vi "test_save_2.vi"() -> ()   [LabVIEW 2016]
panel:
  out "4":i32
  out "3":i32
  out "2":i32
  out "1":i32
  out "4":string
  out "положение 4":i32
  out "3":string
  out "положение 3":i32
  in  "Numeric 4":i32
  in  "Numeric 3":i32
  out "2":string
  out "положение 2":i32
  in  "Numeric 2":i32
  out "положение":i32
  in  "Numeric":i32
  in  "stop":bool
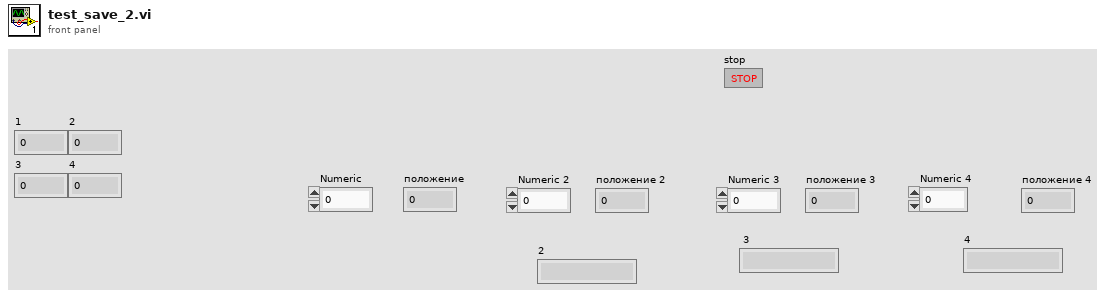
[diagram p1: front panel]
types:
  T1 = enum16{"open", "replace", "create", "open or create", "replace or create", "replace or create with confirmation"}
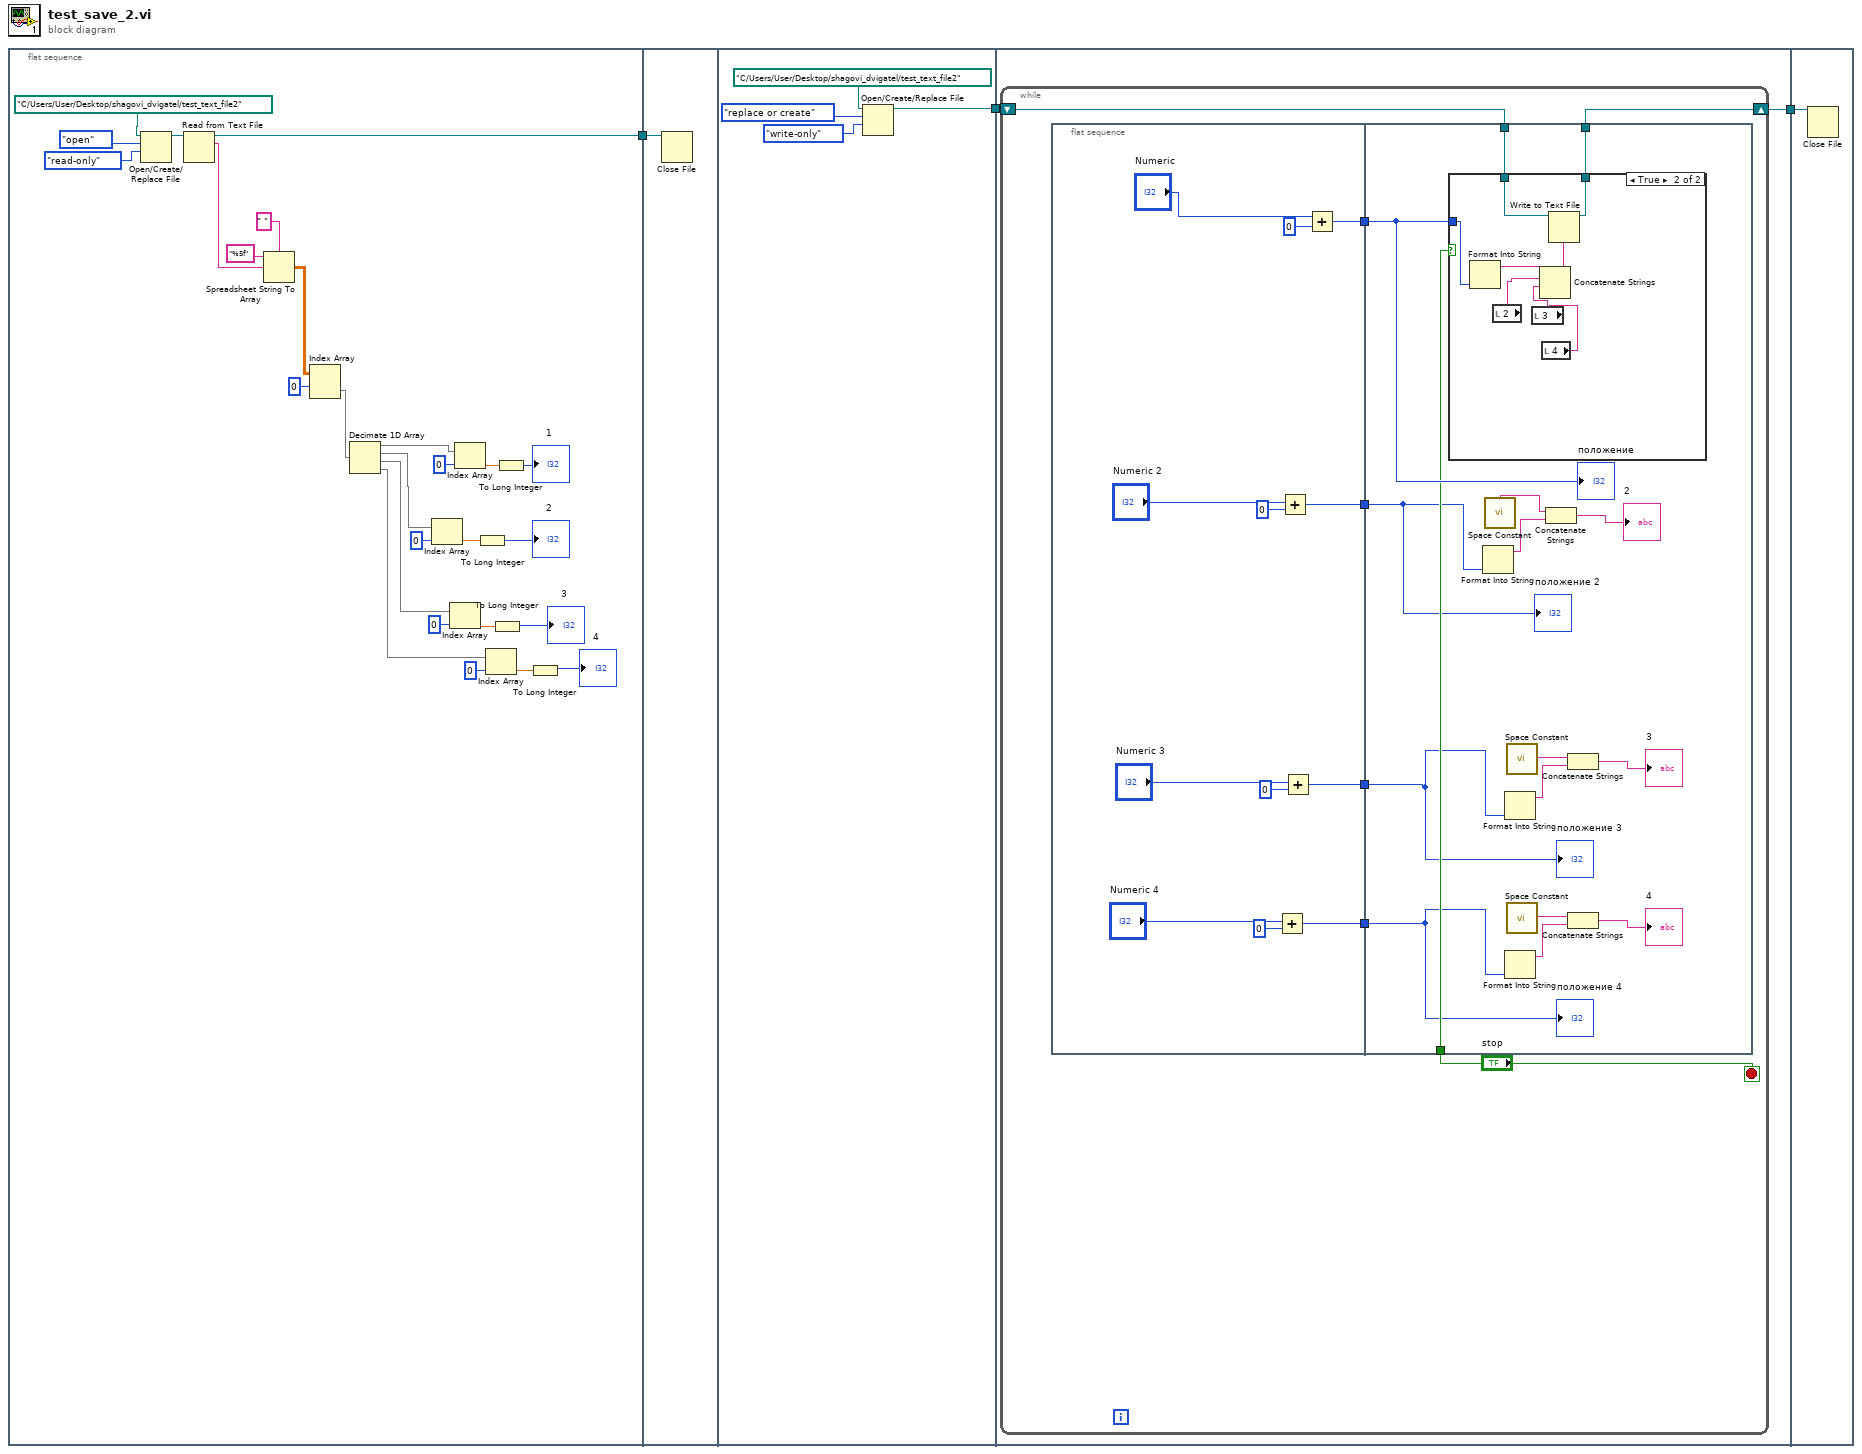
[diagram p0: block diagram]
diagram:
  n1 = flat-sequence {
    tunnel: [w26] -> w3
    tunnel: w3 -> [w31]
    tunnel: [w32] -> w1
    tunnel: [w37] -> w2
    tunnel: w1 -> [w36]
    tunnel: w2 -> [w82]
    frame #0 {
      n2 = Open/Create/Replace File(file path (use dialog)=path "C:/Users/User/Desktop/shagovi_dvigatel/test_text_file2", operation (0:open)=T1."open", access (0:read/write)=enum16{"read/write", "read-only", "write-only"}."read-only") -> (refnum out=w27:refnum<file>)  [unwired: 3 in, 2 out]
      n3 = Read from Text File(file (use dialog)=w27) -> (refnum out=w26:refnum<file>, text=w24:string)  [unwired: 3 in, 2 out]
      n4 = Spreadsheet String To Array(delimiter (Tab)=" ", format string="%5f", spreadsheet string=w24) -> (array=w22:dbl[][])  [unwired: 1 in]
      n5 = Index Array(array=w22, index (row)=0 ("index")) -> (element=w20:dbl[])  [unwired: 1 in]
      n6 = Decimate 1D Array(w20) -> (w12:dbl[], w14:dbl[], w16:dbl[], w19:dbl[])
      n7 = Index Array(array=w14, index=0) -> (element=w9:dbl)
      n8 = Index Array(array=w16, index=0) -> (element=w10:dbl)
      n9 = Index Array(array=w12, index=0) -> (element=w8:dbl)
      n10 = To Long Integer(number=w9) -> (32bit integer=→"2":i32)
      n11 = Index Array(array=w19, index=0) -> (element=w11:dbl)
      n12 = To Long Integer(number=w10) -> (32bit integer=→"3":i32)
      n13 = To Long Integer(number=w8) -> (32bit integer=→"1":i32)
      n14 = To Long Integer(number=w11) -> (32bit integer=→"4":i32)
    }
    frame #1 {
      n15 = Close File(refnum=w31) -> ()  [unwired: 1 in, 2 out]
    }
    frame #2 {
      n16 = Open/Create/Replace File(file path (use dialog)=path "C:/Users/User/Desktop/shagovi_dvigatel/test_text_file2", operation (0:open)=T1."replace or create", access (0:read/write)=enum16{"read/write", "read-only", "write-only"}."write-only") -> (refnum out=w32:refnum<file>)  [unwired: 3 in, 2 out]
    }
    frame #3 {
      n17 = while {
        shift-right: [w44] -> w37
        shift-left: w36 -> [w43]
        stop <- "stop" stop-if-true
        n18 = flat-sequence {
          tunnel: [w55] -> w42
          tunnel: [w53] -> w40
          tunnel: [w46] -> w39
          tunnel: [w45] -> w38
          tunnel: [w72] -> w44
          tunnel: w43 -> [w71]
          tunnel: w42 -> [w70]
          tunnel: "stop" -> [w69]
          tunnel: w40 -> [w68]
          tunnel: w39 -> [w60]
          tunnel: w38 -> [w59]
          frame #0 {
            n19 = Add(x="Numeric 4", y=0) -> (x+y=w46:i32)
            n20 = Add(x="Numeric 2", y=0) -> (x+y=w53:i32)
            n21 = Add(x="Numeric 3", y=0) -> (x+y=w45:i32)
            n22 = Add(x="Numeric", y=0) -> (x+y=w55:i32)
          }
          frame #1 {
            n23 = case shown="True" w69 {
              tunnel: w71 -> [w73 w81]
              tunnel: [w73 w80] -> w72
              tunnel: w70 -> [_ w79]
              frame False {
              }
              frame True {
                n24 = Format Into String(w79) -> (resulting string=w78:string)  [unwired: 3 in, 1 out]
                n25 = local read "2"() -> (w77:string)
                n26 = local read "3"() -> (w75:string)
                n27 = local read "4"() -> (w74:string)
                n28 = Concatenate Strings(w78, w77, w75, w74) -> (w76:string)
                n29 = Write to Text File(file (use dialog)=w81, text=w76) -> (refnum out=w80:refnum<file>)  [unwired: 2 in, 2 out]
              }
            }
            n30 = Format Into String(w68) -> (resulting string=w65:string)  [unwired: 3 in, 1 out]
            n31 = call <vilib>:"Space Constant.vi"() -> ("String"=w66:string)
            n32 = Format Into String(w59) -> (resulting string=w63:string)  [unwired: 3 in, 1 out]
            n33 = Format Into String(w60) -> (resulting string=w61:string)  [unwired: 3 in, 1 out]
            n34 = call <vilib>:"Space Constant.vi"() -> ("String"=w58:string)
            n35 = call <vilib>:"Space Constant.vi"() -> ("String"=w57:string)
            n36 = Concatenate Strings(w66, w65) -> (→"2":string)
            n37 = Concatenate Strings(w58, w63) -> (→"3":string)
            n38 = Concatenate Strings(w57, w61) -> (→"4":string)
            "положение" <- w70
            "положение 2" <- w68
            "положение 3" <- w59
            "положение 4" <- w60
          }
        }
      }
    }
    frame #4 {
      n39 = Close File(refnum=w82) -> ()  [unwired: 1 in, 2 out]
    }
  }
